vi "Perform Action on Target.vi"(8 "error in":errorcluster, 9 "Input":variant, 10 "Task-Point Ident":string, 11 "IStudy Actor in":refnum<class "IStudy Actor.lvclass">) -> (0 "error out":errorcluster, 3 "IStudy Actor out":refnum<class "IStudy Actor.lvclass">)   [LabVIEW 2024, in "IStudy Actor.lvlib" / "IStudy Actor.lvclass"]
uses:
  IStudy Actor.lvclass
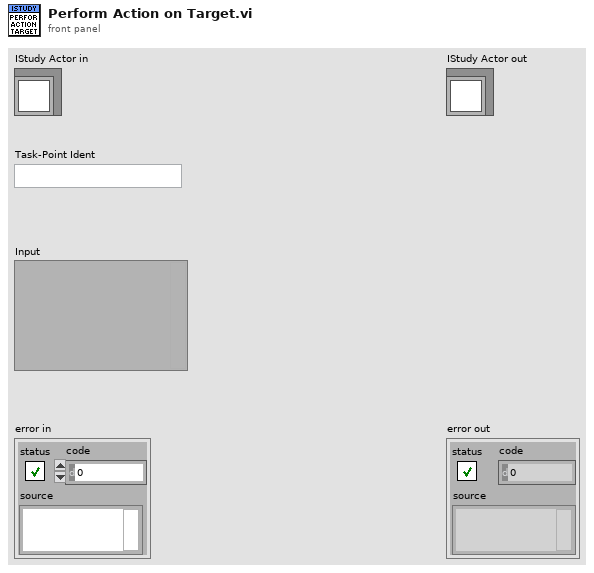
[diagram p1: front panel]
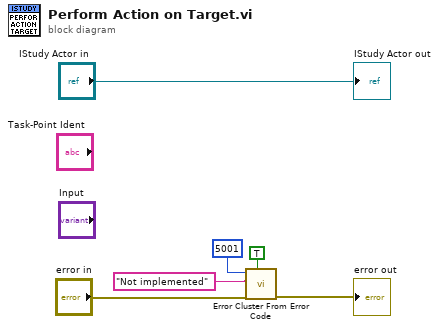
[diagram p0: block diagram]
diagram:
  n1 = call <vilib>:"Error Cluster From Error Code.vi"("show call chain? (False)"=TRUE, "error in (no error)"="error in", "error message (\"\")"="Not implemented" ("error message (\"\")"), "error code (0)"=5001) -> ("error out"=→"error out":errorcluster)  [unwired: 5 in]
  "IStudy Actor out" <- "IStudy Actor in"
